vi "Read LIST_IO.vi"(0 "file (use dialog)":path) -> (11 "IP":string, 15 "MERKER":T2, 18 "DATABLOCK":T1)   [LabVIEW 2019]
uses:
  <vilib>/Utility/file.llb/Read Delimited Spreadsheet (string).vi
panel:
  out "all rows":string[][](array[string])
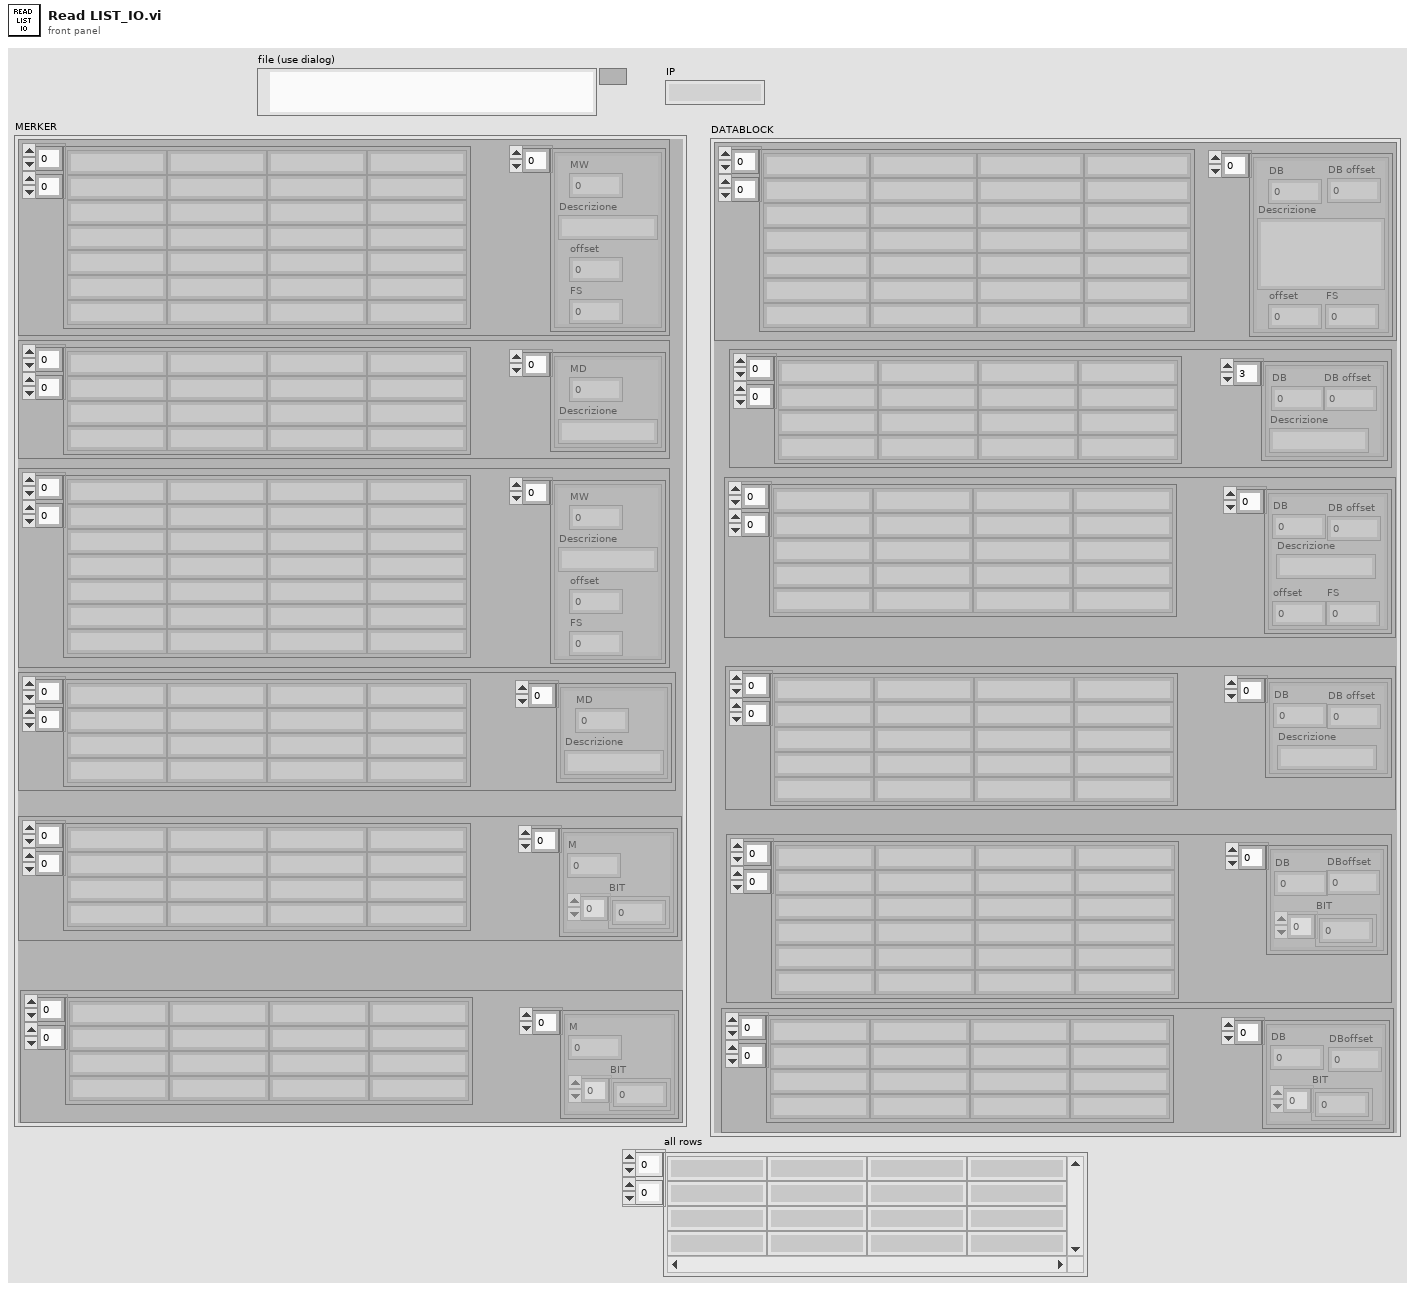
[diagram p1: front panel]
types:
  T1 = cluster{cluster{string[][], cluster{"DB":i16, "DB offset":i16, "Descrizione":string, "offset":dbl, "FS":dbl}[]}, cluster{string[][], cluster{"DB":i16, "Descrizione":string, "DB offset":i16}[]}, cluster{string[][], cluster{"DB":i16, "DB offset":i16, "Descrizione":string, "offset":dbl, "FS":dbl}[]}, cluster{string[][], cluster{"DB":i16, "Descrizione":string, "DB offset":i16}[]}, cluster{string[][], cluster{"DB":i16, "BIT":i16[], "DBoffset":i16}[]}, cluster{string[][], cluster{"DB":i16, "BIT":i16[], "DBoffset":i16}[]}}
  T2 = cluster{cluster{string[][], cluster{"MW":dbl, "Descrizione":string, "offset":dbl, "FS":dbl}[]}, cluster{string[][], cluster{"MD":i16, "Descrizione":string}[]}, cluster{string[][], cluster{"MW":dbl, "Descrizione":string, "offset":dbl, "FS":dbl}[]}, cluster{string[][], cluster{"MD":i16, "Descrizione":string}[]}, cluster{string[][], cluster{"M":i16, "BIT":i16[]}[]}, cluster{string[][], cluster{"M":i16, "BIT":i16[]}[]}}
  T3 = cluster{"DB":i16, "Descrizione":string, "DB offset":i16}
  T4 = cluster{"DB":i16, "DB offset":i16, "Descrizione":string, "offset":dbl, "FS":dbl}
  T5 = cluster{"MW":dbl, "Descrizione":string, "offset":dbl, "FS":dbl}
  T6 = cluster{"DB":i16, "Descrizione":string, "DB offset":i16}[]
  T7 = cluster{string[][], cluster{"MW":dbl, "Descrizione":string, "offset":dbl, "FS":dbl}[]}
  T8 = cluster{string[][], cluster{"MD":i16, "Descrizione":string}[]}
  T9 = cluster{string[][], cluster{"M":i16, "BIT":i16[]}[]}
  T10 = cluster{string[][], cluster{"DB":i16, "BIT":i16[], "DBoffset":i16}[]}
  T11 = cluster{string[][], cluster{"DB":i16, "DB offset":i16, "Descrizione":string, "offset":dbl, "FS":dbl}[]}
  T12 = cluster{string[][], cluster{"DB":i16, "Descrizione":string, "DB offset":i16}[]}
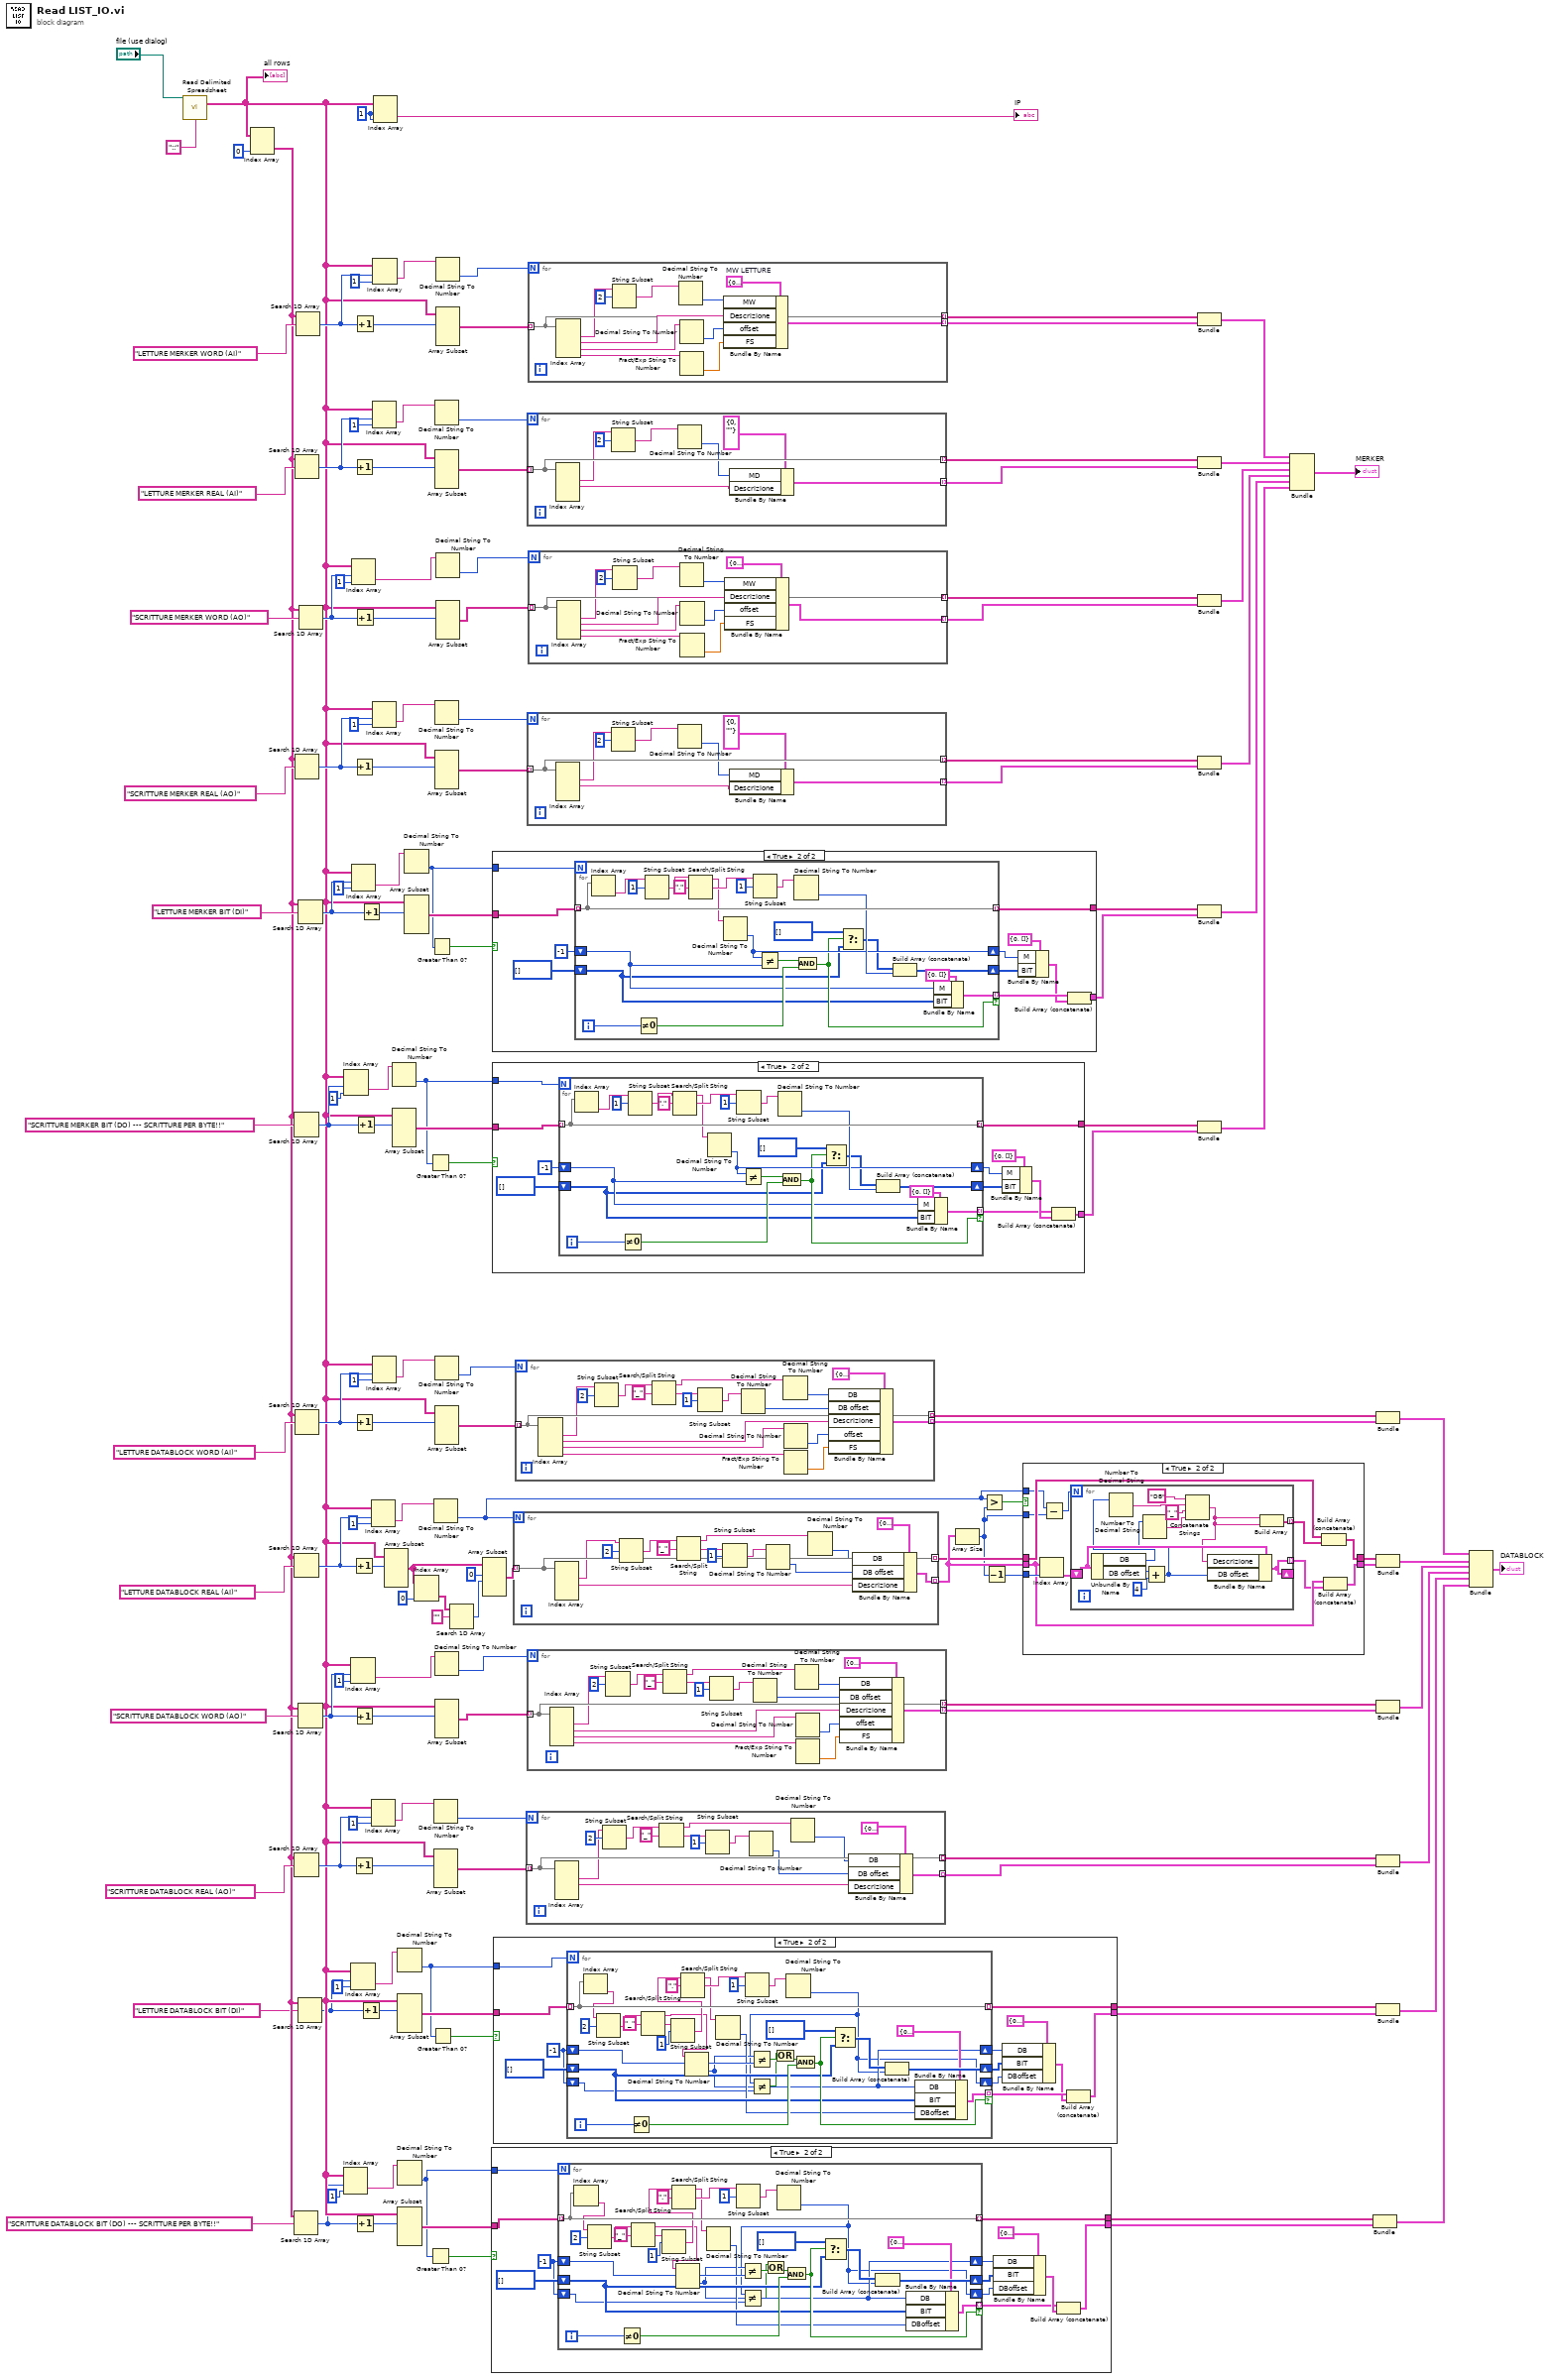
[diagram p0: block diagram]
diagram:
  w115 = 1 ("index (row)")
  n1 = call-poly <vilib>:"Read Delimited Spreadsheet.vi"("file path (dialog if empty)"="file (use dialog)", "delimiter (\\t)"="::" ("delimiter (\\t)")) -> ("all rows"=w45:string[][])  [unwired: 8 in, 5 out]
  "all rows" <- w45
  n2 = Index Array(array=w45, index (col)=0 ("disabled index (col)")) -> (element=w46:string[])  [unwired: 1 in]
  n3 = Search 1D Array(1D array=w46, element="SCRITTURE DATABLOCK BIT (DO) --- SCRITTURE PER BYTE!!") -> (index of element=w36:i32)  [unwired: 1 in]
  n4 = Search 1D Array(1D array=w46, element="SCRITTURE MERKER BIT (DO) --- SCRITTURE PER BYTE!!") -> (index of element=w118:i32)  [unwired: 1 in]
  n5 = Search 1D Array(1D array=w46, element="LETTURE DATABLOCK REAL (AI)") -> (index of element=w62:i32)  [unwired: 1 in]
  n6 = Search 1D Array(1D array=w46, element="SCRITTURE DATABLOCK REAL (AO)") -> (index of element=w65:i32)  [unwired: 1 in]
  n7 = Search 1D Array(1D array=w46, element="LETTURE MERKER REAL (AI)") -> (index of element=w108:i32)  [unwired: 1 in]
  n8 = Search 1D Array(1D array=w46, element="SCRITTURE MERKER REAL (AO)") -> (index of element=w105:i32)  [unwired: 1 in]
  n9 = Search 1D Array(1D array=w46, element="LETTURE DATABLOCK WORD (AI)") -> (index of element=w51:i32)  [unwired: 1 in]
  n10 = Search 1D Array(1D array=w46, element="LETTURE MERKER WORD (AI)") -> (index of element=w133:i32)  [unwired: 1 in]
  n11 = Search 1D Array(1D array=w46, element="LETTURE DATABLOCK BIT (DI)") -> (index of element=w33:i32)  [unwired: 1 in]
  n12 = Search 1D Array(1D array=w46, element="LETTURE MERKER BIT (DI)") -> (index of element=w121:i32)  [unwired: 1 in]
  n13 = Search 1D Array(1D array=w46, element="SCRITTURE DATABLOCK WORD (AO)") -> (index of element=w56:i32)  [unwired: 1 in]
  n14 = Search 1D Array(1D array=w46, element="SCRITTURE MERKER WORD (AO)") -> (index of element=w128:i32)  [unwired: 1 in]
  n15 = Index Array(array=w45, index (row)=w36, index (col)=1 ("disabled index (col)")) -> (element=w35:string)
  n16 = Index Array(array=w45, index (row)=w118, index (col)=1 ("disabled index (col)")) -> (element=w119:string)
  n17 = Index Array(array=w45, index (row)=w56, index (col)=1 ("disabled index (col)")) -> (element=w58:string)
  n18 = Index Array(array=w45, index (row)=w33, index (col)=1 ("disabled index (col)")) -> (element=w31:string)
  n19 = Index Array(array=w45, index (row)=w128, index (col)=1 ("disabled index (col)")) -> (element=w126:string)
  n20 = Index Array(array=w45, index (row)=w121, index (col)=1 ("disabled index (col)")) -> (element=w123:string)
  n21 = Increment(x=w62) -> (x+1=w63:i32)
  n22 = Increment(x=w65) -> (x+1=w64:i32)
  n23 = Increment(x=w108) -> (x+1=w107:i32)
  n24 = Increment(x=w105) -> (x+1=w106:i32)
  n25 = Increment(x=w51) -> (x+1=w54:i32)
  n26 = Increment(x=w56) -> (x+1=w49:i32)
  n27 = Increment(x=w133) -> (x+1=w130:i32)
  n28 = Increment(x=w128) -> (x+1=w140:i32)
  n29 = Increment(x=w36) -> (x+1=w29:i32)
  n30 = Increment(x=w118) -> (x+1=w137:i32)
  n31 = Increment(x=w33) -> (x+1=w34:i32)
  n32 = Increment(x=w121) -> (x+1=w120:i32)
  n33 = Index Array(array=w45, index (row)=w62, index (col)=1 ("disabled index (row)")) -> (element=w60:string)
  n34 = Index Array(array=w45, index (row)=w65, index (col)=1 ("disabled index (row)")) -> (element=w67:string)
  n35 = Index Array(array=w45, index (row)=w108, index (col)=1 ("disabled index (row)")) -> (element=w110:string)
  n36 = Index Array(array=w45, index (row)=w105, index (col)=1 ("disabled index (row)")) -> (element=w103:string)
  n37 = Index Array(array=w45, index (row)=w51, index (col)=1 ("disabled index (row)")) -> (element=w50:string)
  n38 = Index Array(array=w45, index (row)=w133, index (col)=1 ("disabled index (row)")) -> (element=w134:string)
  n39 = Index Array(array=w45, index (row)=w115, index (col)=w115) -> (element=→"IP":string)
  n40 = Array Subset(array=w45, index (row)=w63) -> (w5:string[][])  [unwired: 3 in]
  n41 = Decimal String To Number(string=w119) -> (number=w21:i32)  [unwired: 2 in, 1 out]
  n42 = Array Subset(array=w45, index (row)=w137) -> (w116:string[][])  [unwired: 3 in]
  n43 = Decimal String To Number(string=w31) -> (number=w18:i32)  [unwired: 2 in, 1 out]
  n44 = Array Subset(array=w45, index (row)=w34) -> (w28:string[][])  [unwired: 3 in]
  n45 = Decimal String To Number(string=w35) -> (number=w17:i32)  [unwired: 2 in, 1 out]
  n46 = Array Subset(array=w45, index (row)=w29) -> (w24:string[][])  [unwired: 3 in]
  n47 = Decimal String To Number(string=w123) -> (number=w22:i32)  [unwired: 2 in, 1 out]
  n48 = Array Subset(array=w45, index (row)=w120) -> (w138:string[][])  [unwired: 3 in]
  n49 = Index Array(array=w5, index (col)=0 ("disabled index (col)")) -> (element=w8:string[])  [unwired: 1 in]
  n50 = Greater Than 0?(x=w21) -> (x > 0?=w20:bool)
  n51 = Greater Than 0?(x=w17) -> (x > 0?=w16:bool)
  n52 = Greater Than 0?(x=w22) -> (x > 0?=w23:bool)
  n53 = Greater Than 0?(x=w18) -> (x > 0?=w19:bool)
  n54 = Decimal String To Number(string=w60) -> (number=w10:i32)  [unwired: 2 in, 1 out]
  n55 = Decimal String To Number(string=w67) -> (number=w69:i32)  [unwired: 2 in, 1 out]
  n56 = Array Subset(array=w45, index (row)=w64) -> (w70:string[][])  [unwired: 3 in]
  n57 = Decimal String To Number(string=w110) -> (number=w112:i32)  [unwired: 2 in, 1 out]
  n58 = Array Subset(array=w45, index (row)=w107) -> (w113:string[][])  [unwired: 3 in]
  n59 = Decimal String To Number(string=w103) -> (number=w101:i32)  [unwired: 2 in, 1 out]
  n60 = Array Subset(array=w45, index (row)=w106) -> (w100:string[][])  [unwired: 3 in]
  n61 = Decimal String To Number(string=w50) -> (number=w53:i32)  [unwired: 2 in, 1 out]
  n62 = Array Subset(array=w45, index (row)=w54) -> (w55:string[][])  [unwired: 3 in]
  n63 = Decimal String To Number(string=w58) -> (number=w44:i32)  [unwired: 2 in, 1 out]
  n64 = Array Subset(array=w45, index (row)=w49) -> (w43:string[][])  [unwired: 3 in]
  n65 = Decimal String To Number(string=w134) -> (number=w131:i32)  [unwired: 2 in, 1 out]
  n66 = Array Subset(array=w45, index (row)=w130) -> (w129:string[][])  [unwired: 3 in]
  n67 = Decimal String To Number(string=w126) -> (number=w124:i32)  [unwired: 2 in, 1 out]
  n68 = Array Subset(array=w45, index (row)=w140) -> (w125:string[][])  [unwired: 3 in]
  n69 = Search 1D Array(1D array=w8, element="") -> (index of element=w2:i32)  [unwired: 1 in]
  n70 = Array Subset(array=w5, index (row)=0 ("index"), length (row)=w2) -> (w4:string[][])  [unwired: 2 in]
  n71 = case shown="True" w16 {
    tunnel: [_ w151] -> w26
    tunnel: [_ w150] -> w25
    tunnel: w17 -> [_ w149]
    tunnel: w24 -> [_ w148]
    frame False {
    }
    frame True {
      w147 = -1 ("offset past number")
      n72 = for {
        N: w149 -> [_]
        tunnel: w148 -> [w187] mode=indexing
        tunnel: [w187] -> w151 mode=indexing
        shift-right: [w161] -> w155
        shift-left: w147 -> [w176]
        shift-right: [w174] -> w146
        shift-left: i32[] [] ("BIT") -> [w173]
        tunnel: [w181] -> w152 mode=indexing if=w179
        shift-right: [w159] -> w145
        shift-left: w147 -> [w160]
        i -> [w177]
        n73 = Index Array(array=w187) -> (element=w166:string)  [unwired: 1 in]
        n74 = String Subset(string=w166, offset (0)=2) -> (substring=w171:string)  [unwired: 1 in]
        n75 = Not Equal To 0?(x=w177) -> (x != 0?=w178:bool)
        n76 = Search/Split String(string=w171, search string/char (-)="_") -> (substring before match=w162:string, match + rest of string=w169:string)  [unwired: 1 in, 1 out]
        n77 = String Subset(string=w169, offset (0)=1) -> (substring=w165:string)  [unwired: 1 in]
        n78 = Search/Split String(string=w165, search string/char (-)=".") -> (substring before match=w182:string, match + rest of string=w184:string)  [unwired: 1 in, 1 out]
        n79 = Decimal String To Number(string=w162) -> (number=w161:i32)  [unwired: 2 in, 1 out]
        n80 = Decimal String To Number(string=w182) -> (number=w163:i32)  [unwired: 2 in, 1 out]
        n81 = String Subset(string=w184, offset (0)=1) -> (substring=w183:string)  [unwired: 1 in]
        n82 = Not Equal?(x=w161, y=w176) -> (x != y?=w175:bool)
        n83 = Decimal String To Number(string=w183) -> (number=w159:i32)  [unwired: 2 in, 1 out]
        n84 = Not Equal?(x=w159, y=w160) -> (x != y?=w157:bool)
        n85 = Or(x=w157, y=w175) -> (x .or. y?=w158:bool)
        n86 = And(x=w158, y=w178) -> (x .and. y?=w179:bool)
        n87 = Select(t=i16[] [] ("BIT"), s=w179, f=w173) -> (s? t:f=w172:i32[])
        n88 = Build Array (concatenate)(w172, w159) -> (w174:i32[])
        n89 = Bundle By Name(cluster=cluster{"DB":i16, "BIT":i16[], "DBoffset":i16} {"DB"=0, "BIT"=[], "DBoffset"=0} ("M BIT LETTURE"), "DB"=w161, "BIT"=w173, "DBoffset"=w163) -> (w181:cluster{"DB":i16, "BIT":i16[], "DBoffset":i16})
      }
      n90 = Bundle By Name(cluster=cluster{"DB":i16, "BIT":i16[], "DBoffset":i16} {"DB"=0, "BIT"=[], "DBoffset"=0} ("M BIT LETTURE"), "DB"=w155, "BIT"=w146, "DBoffset"=w145) -> (w156:cluster{"DB":i16, "BIT":i16[], "DBoffset":i16})
      n91 = Build Array (concatenate)(w152, w156) -> (w150:cluster{"DB":i16, "BIT":i16[], "DBoffset":i16}[])
    }
  }
  n92 = case shown="True" w23 {
    tunnel: w138 -> [_ w198]
    tunnel: w22 -> [_ w197]
    tunnel: [_ w189] -> w91
    tunnel: [_ w188] -> w90
    frame False {
    }
    frame True {
      n93 = for {
        N: w197 -> [_]
        tunnel: w198 -> [w220] mode=indexing
        tunnel: [w220] -> w189 mode=indexing
        shift-right: [w207] -> w193
        shift-left: -1 ("offset past number") -> [w203]
        shift-right: [w201] -> w192
        shift-left: i32[] [] ("BIT") -> [w200]
        tunnel: [w210] -> w191 mode=indexing if=w206
        i -> [w204]
        n94 = Index Array(array=w220) -> (element=w218:string)  [unwired: 1 in]
        n95 = Not Equal To 0?(x=w204) -> (x != 0?=w205:bool)
        n96 = String Subset(string=w218, offset (0)=1) -> (substring=w216:string)  [unwired: 1 in]
        n97 = Search/Split String(string=w216, search string/char (-)=".") -> (substring before match=w212:string, match + rest of string=w214:string)  [unwired: 1 in, 1 out]
        n98 = Decimal String To Number(string=w212) -> (number=w207:i32)  [unwired: 2 in, 1 out]
        n99 = String Subset(string=w214, offset (0)=1) -> (substring=w213:string)  [unwired: 1 in]
        n100 = Not Equal?(x=w207, y=w203) -> (x != y?=w202:bool)
        n101 = Decimal String To Number(string=w213) -> (number=w208:i32)  [unwired: 2 in, 1 out]
        n102 = And(x=w202, y=w205) -> (x .and. y?=w206:bool)
        n103 = Select(t=i16[] [] ("BIT"), s=w206, f=w200) -> (s? t:f=w199:i32[])
        n104 = Build Array (concatenate)(w199, w208) -> (w201:i32[])
        n105 = Bundle By Name(cluster=cluster{"M":i16, "BIT":i16[]} {"M"=0, "BIT"=[]} ("M BIT LETTURE"), "M"=w203, "BIT"=w200) -> (w210:cluster{"M":i16, "BIT":i16[]})
      }
      n106 = Bundle By Name(cluster=cluster{"M":i16, "BIT":i16[]} {"M"=0, "BIT"=[]} ("M BIT LETTURE"), "M"=w193, "BIT"=w192) -> (w190:cluster{"M":i16, "BIT":i16[]})
      n107 = Build Array (concatenate)(w191, w190) -> (w188:cluster{"M":i16, "BIT":i16[]}[])
    }
  }
  n108 = case shown="True" w20 {
    tunnel: w21 -> [_ w224]
    tunnel: w116 -> [_ w223]
    tunnel: [_ w222] -> w89
    tunnel: [_ w221] -> w88
    frame False {
    }
    frame True {
      n109 = for {
        N: w224 -> [_]
        tunnel: w223 -> [w253] mode=indexing
        tunnel: [w253] -> w222 mode=indexing
        shift-right: [w240] -> w228
        shift-left: -1 ("offset past number") -> [w236]
        shift-right: [w234] -> w229
        shift-left: i32[] [] ("BIT") -> [w233]
        tunnel: [w243] -> w230 mode=indexing if=w239
        i -> [w237]
        n110 = Index Array(array=w253) -> (element=w251:string)  [unwired: 1 in]
        n111 = Not Equal To 0?(x=w237) -> (x != 0?=w238:bool)
        n112 = String Subset(string=w251, offset (0)=1) -> (substring=w249:string)  [unwired: 1 in]
        n113 = Search/Split String(string=w249, search string/char (-)=".") -> (substring before match=w245:string, match + rest of string=w247:string)  [unwired: 1 in, 1 out]
        n114 = Decimal String To Number(string=w245) -> (number=w240:i32)  [unwired: 2 in, 1 out]
        n115 = String Subset(string=w247, offset (0)=1) -> (substring=w246:string)  [unwired: 1 in]
        n116 = Not Equal?(x=w240, y=w236) -> (x != y?=w235:bool)
        n117 = Decimal String To Number(string=w246) -> (number=w241:i32)  [unwired: 2 in, 1 out]
        n118 = And(x=w235, y=w238) -> (x .and. y?=w239:bool)
        n119 = Select(t=i16[] [] ("BIT"), s=w239, f=w233) -> (s? t:f=w232:i32[])
        n120 = Build Array (concatenate)(w232, w241) -> (w234:i32[])
        n121 = Bundle By Name(cluster=cluster{"M":i16, "BIT":i16[]} {"M"=0, "BIT"=[]} ("M BIT LETTURE"), "M"=w236, "BIT"=w233) -> (w243:cluster{"M":i16, "BIT":i16[]})
      }
      n122 = Bundle By Name(cluster=cluster{"M":i16, "BIT":i16[]} {"M"=0, "BIT"=[]} ("M BIT LETTURE"), "M"=w228, "BIT"=w229) -> (w231:cluster{"M":i16, "BIT":i16[]})
      n123 = Build Array (concatenate)(w230, w231) -> (w221:cluster{"M":i16, "BIT":i16[]}[])
    }
  }
  n124 = case shown="True" w19 {
    tunnel: [_ w265] -> w39
    tunnel: [_ w264] -> w38
    tunnel: w18 -> [_ w261]
    tunnel: w28 -> [_ w260]
    frame False {
    }
    frame True {
      w259 = -1 ("offset past number")
      n125 = for {
        N: w261 -> [_]
        tunnel: w260 -> [w296] mode=indexing
        tunnel: [w296] -> w264 mode=indexing
        shift-right: [w270] -> w257
        shift-left: w259 -> [w285]
        shift-right: [w283] -> w256
        shift-left: i32[] [] ("BIT") -> [w282]
        tunnel: [w290] -> w263 mode=indexing if=w288
        shift-right: [w268] -> w255
        shift-left: w259 -> [w269]
        i -> [w286]
        n126 = Index Array(array=w296) -> (element=w275:string)  [unwired: 1 in]
        n127 = String Subset(string=w275, offset (0)=2) -> (substring=w280:string)  [unwired: 1 in]
        n128 = Not Equal To 0?(x=w286) -> (x != 0?=w287:bool)
        n129 = Search/Split String(string=w280, search string/char (-)="_") -> (substring before match=w271:string, match + rest of string=w278:string)  [unwired: 1 in, 1 out]
        n130 = String Subset(string=w278, offset (0)=1) -> (substring=w274:string)  [unwired: 1 in]
        n131 = Search/Split String(string=w274, search string/char (-)=".") -> (substring before match=w291:string, match + rest of string=w293:string)  [unwired: 1 in, 1 out]
        n132 = Decimal String To Number(string=w271) -> (number=w270:i32)  [unwired: 2 in, 1 out]
        n133 = Decimal String To Number(string=w291) -> (number=w272:i32)  [unwired: 2 in, 1 out]
        n134 = String Subset(string=w293, offset (0)=1) -> (substring=w292:string)  [unwired: 1 in]
        n135 = Not Equal?(x=w270, y=w285) -> (x != y?=w284:bool)
        n136 = Decimal String To Number(string=w292) -> (number=w268:i32)  [unwired: 2 in, 1 out]
        n137 = Not Equal?(x=w268, y=w269) -> (x != y?=w266:bool)
        n138 = Or(x=w266, y=w284) -> (x .or. y?=w267:bool)
        n139 = And(x=w267, y=w287) -> (x .and. y?=w288:bool)
        n140 = Select(t=i16[] [] ("BIT"), s=w288, f=w282) -> (s? t:f=w281:i32[])
        n141 = Build Array (concatenate)(w281, w268) -> (w283:i32[])
        n142 = Bundle By Name(cluster=cluster{"DB":i16, "BIT":i16[], "DBoffset":i16} {"DB"=0, "BIT"=[], "DBoffset"=0} ("M BIT LETTURE"), "DB"=w270, "BIT"=w282, "DBoffset"=w272) -> (w290:cluster{"DB":i16, "BIT":i16[], "DBoffset":i16})
      }
      n143 = Bundle By Name(cluster=cluster{"DB":i16, "BIT":i16[], "DBoffset":i16} {"DB"=0, "BIT"=[], "DBoffset"=0} ("M BIT LETTURE"), "DB"=w257, "BIT"=w256, "DBoffset"=w255) -> (w254:cluster{"DB":i16, "BIT":i16[], "DBoffset":i16})
      n144 = Build Array (concatenate)(w263, w254) -> (w265:cluster{"DB":i16, "BIT":i16[], "DBoffset":i16}[])
    }
  }
  n145 = for {
    N: w10 -> [_]
    tunnel: [w310] -> w12 mode=indexing
    tunnel: w4 -> [w310] mode=indexing
    tunnel: [w308] -> w14 mode=indexing
    n146 = Index Array(array=w310) -> (element #1=w299:string, element #2=w309:string)  [unwired: 4 in, 2 out]
    n147 = String Subset(string=w299, offset (0)=2) -> (substring=w301:string)  [unwired: 1 in]
    n148 = Search/Split String(string=w301, search string/char (-)="_") -> (substring before match=w302:string, match + rest of string=w304:string)  [unwired: 1 in, 1 out]
    n149 = String Subset(string=w304, offset (0)=1) -> (substring=w306:string)  [unwired: 1 in]
    n150 = Decimal String To Number(string=w306) -> (number=w297:i32)  [unwired: 2 in, 1 out]
    n151 = Decimal String To Number(string=w302) -> (number=w298:i32)  [unwired: 2 in, 1 out]
    n152 = Bundle By Name(cluster=T3 {"DB"=0, "Descrizione"="", "DB offset"=0} ("MW LETTURE 2"), "DB"=w298, "DB offset"=w297, "Descrizione"=w309) -> (w308:T3)
  }
  n153 = for {
    N: w53 -> [_]
    tunnel: [w322] -> w71 mode=indexing
    tunnel: [w323] -> w72 mode=indexing
    tunnel: w55 -> [w322] mode=indexing
    n154 = Index Array(array=w322) -> (element #1=w321:string, element #2=w328:string, element #3=w327:string, element #4=w325:string)  [unwired: 4 in]
    n155 = String Subset(string=w321, offset (0)=2) -> (substring=w319:string)  [unwired: 1 in]
    n156 = Search/Split String(string=w319, search string/char (-)="_") -> (substring before match=w318:string, match + rest of string=w316:string)  [unwired: 1 in, 1 out]
    n157 = String Subset(string=w316, offset (0)=1) -> (substring=w314:string)  [unwired: 1 in]
    n158 = Decimal String To Number(string=w314) -> (number=w312:i32)  [unwired: 2 in, 1 out]
    n159 = Decimal String To Number(string=w318) -> (number=w313:i32)  [unwired: 2 in, 1 out]
    n160 = Decimal String To Number(string=w327) -> (number=w326:i32)  [unwired: 2 in, 1 out]
    n161 = Fract/Exp String To Number(string=w325) -> (number=w324:dbl)  [unwired: 3 in, 1 out]
    n162 = Bundle By Name(cluster=T4 {"DB"=0, "DB offset"=0, "Descrizione"="", "offset"=0.0, "FS"=0.0} ("MW LETTURE 2"), "DB"=w313, "DB offset"=w312, "Descrizione"=w328, "offset"=w326, "FS"=w324) -> (w323:T4)
  }
  n163 = for {
    N: w69 -> [_]
    tunnel: [w342] -> w73 mode=indexing
    tunnel: w70 -> [w342] mode=indexing
    tunnel: [w340] -> w74 mode=indexing
    n164 = Index Array(array=w342) -> (element #1=w332:string, element #2=w341:string)  [unwired: 4 in, 2 out]
    n165 = String Subset(string=w332, offset (0)=2) -> (substring=w334:string)  [unwired: 1 in]
    n166 = Search/Split String(string=w334, search string/char (-)="_") -> (substring before match=w335:string, match + rest of string=w337:string)  [unwired: 1 in, 1 out]
    n167 = String Subset(string=w337, offset (0)=1) -> (substring=w339:string)  [unwired: 1 in]
    n168 = Decimal String To Number(string=w339) -> (number=w329:i32)  [unwired: 2 in, 1 out]
    n169 = Decimal String To Number(string=w335) -> (number=w330:i32)  [unwired: 2 in, 1 out]
    n170 = Bundle By Name(cluster=T3 {"DB"=0, "Descrizione"="", "DB offset"=0} ("MW LETTURE 2"), "DB"=w330, "DB offset"=w329, "Descrizione"=w341) -> (w340:T3)
  }
  n171 = for {
    N: w112 -> [_]
    tunnel: [w350] -> w97 mode=indexing
    tunnel: w113 -> [w350] mode=indexing
    tunnel: [w343] -> w96 mode=indexing
    n172 = Index Array(array=w350) -> (element #1=w349:string, element #2=w344:string)  [unwired: 4 in, 2 out]
    n173 = String Subset(string=w349, offset (0)=2) -> (substring=w347:string)  [unwired: 1 in]
    n174 = Decimal String To Number(string=w347) -> (number=w345:i32)  [unwired: 2 in, 1 out]
    n175 = Bundle By Name(cluster=cluster{"MD":i16, "Descrizione":string} {"MD"=0, "Descrizione"=""} ("MW LETTURE 2"), "MD"=w345, "Descrizione"=w344) -> (w343:cluster{"MD":i16, "Descrizione":string})
  }
  n176 = for {
    N: w101 -> [_]
    tunnel: [w358] -> w93 mode=indexing
    tunnel: w100 -> [w358] mode=indexing
    tunnel: [w351] -> w92 mode=indexing
    n177 = Index Array(array=w358) -> (element #1=w357:string, element #2=w352:string)  [unwired: 4 in, 2 out]
    n178 = String Subset(string=w357, offset (0)=2) -> (substring=w355:string)  [unwired: 1 in]
    n179 = Decimal String To Number(string=w355) -> (number=w353:i32)  [unwired: 2 in, 1 out]
    n180 = Bundle By Name(cluster=cluster{"MD":i16, "Descrizione":string} {"MD"=0, "Descrizione"=""} ("MW LETTURE 2"), "MD"=w353, "Descrizione"=w352) -> (w351:cluster{"MD":i16, "Descrizione":string})
  }
  n181 = for {
    N: w44 -> [_]
    tunnel: [w370] -> w42 mode=indexing
    tunnel: [w371] -> w41 mode=indexing
    tunnel: w43 -> [w370] mode=indexing
    n182 = Index Array(array=w370) -> (element #1=w369:string, element #2=w376:string, element #3=w375:string, element #4=w373:string)  [unwired: 4 in]
    n183 = String Subset(string=w369, offset (0)=2) -> (substring=w367:string)  [unwired: 1 in]
    n184 = Search/Split String(string=w367, search string/char (-)="_") -> (substring before match=w366:string, match + rest of string=w364:string)  [unwired: 1 in, 1 out]
    n185 = String Subset(string=w364, offset (0)=1) -> (substring=w362:string)  [unwired: 1 in]
    n186 = Decimal String To Number(string=w362) -> (number=w360:i32)  [unwired: 2 in, 1 out]
    n187 = Decimal String To Number(string=w366) -> (number=w361:i32)  [unwired: 2 in, 1 out]
    n188 = Decimal String To Number(string=w375) -> (number=w374:i32)  [unwired: 2 in, 1 out]
    n189 = Fract/Exp String To Number(string=w373) -> (number=w372:dbl)  [unwired: 3 in, 1 out]
    n190 = Bundle By Name(cluster=T4 {"DB"=0, "DB offset"=0, "Descrizione"="", "offset"=0.0, "FS"=0.0} ("MW LETTURE 2"), "DB"=w361, "DB offset"=w360, "Descrizione"=w376, "offset"=w374, "FS"=w372) -> (w371:T4)
  }
  n191 = for {
    N: w131 -> [_]
    tunnel: [w380] -> w99 mode=indexing
    tunnel: [w381] -> w98 mode=indexing
    tunnel: w129 -> [w380] mode=indexing
    w388 = T5 {"MW"=0.0, "Descrizione"="", "offset"=0.0, "FS"=0.0}  # MW LETTURE
    n192 = Index Array(array=w380) -> (element #1=w379:string, element #2=w386:string, element #3=w385:string, element #4=w383:string)  [unwired: 4 in]
    n193 = String Subset(string=w379, offset (0)=2) -> (substring=w377:string)  [unwired: 1 in]
    n194 = Decimal String To Number(string=w377) -> (number=w387:i32)  [unwired: 2 in, 1 out]
    n195 = Decimal String To Number(string=w385) -> (number=w384:i32)  [unwired: 2 in, 1 out]
    n196 = Fract/Exp String To Number(string=w383) -> (number=w382:dbl)  [unwired: 3 in, 1 out]
    n197 = Bundle By Name(cluster=w388, "MW"=w387, "Descrizione"=w386, "offset"=w384, "FS"=w382) -> (w381:T5)
  }
  n198 = for {
    N: w124 -> [_]
    tunnel: [w392] -> w95 mode=indexing
    tunnel: [w393] -> w94 mode=indexing
    tunnel: w125 -> [w392] mode=indexing
    n199 = Index Array(array=w392) -> (element #1=w391:string, element #2=w398:string, element #3=w397:string, element #4=w395:string)  [unwired: 4 in]
    n200 = String Subset(string=w391, offset (0)=2) -> (substring=w389:string)  [unwired: 1 in]
    n201 = Decimal String To Number(string=w389) -> (number=w399:i32)  [unwired: 2 in, 1 out]
    n202 = Decimal String To Number(string=w397) -> (number=w396:i32)  [unwired: 2 in, 1 out]
    n203 = Fract/Exp String To Number(string=w395) -> (number=w394:dbl)  [unwired: 3 in, 1 out]
    n204 = Bundle By Name(cluster=T5 {"MW"=0.0, "Descrizione"="", "offset"=0.0, "FS"=0.0} ("MW LETTURE"), "MW"=w399, "Descrizione"=w398, "offset"=w396, "FS"=w394) -> (w393:T5)
  }
  n205 = Array Size(array=w14) -> (size(s)=w9:i32)
  n206 = Greater?(x=w10, y=w9) -> (0:w15:bool)
  n207 = Decrement(x=w9) -> (x-1=w1:i32)
  n208 = case shown="True" w15 {
    tunnel: w14 -> [w401 w411]
    tunnel: w1 -> [_ w413]
    tunnel: [w401 w409] -> w13
    tunnel: w12 -> [w402 w408]
    tunnel: [w402 w406] -> w11
    tunnel: w10 -> [_ w405]
    tunnel: w9 -> [_ w404]
    frame False {
    }
    frame True {
      n209 = Index Array(array=w411, index=w413) -> (element=w412:T3)
      n210 = Subtract(x=w405, y=w404) -> (x-y=w403:i32)
      n211 = for {
        N: w403 -> [_]
        shift-right: [w417] -> _
        shift-left: w412 -> [w425]
        tunnel: [w416] -> w407 mode=indexing
        tunnel: [w417] -> w410 mode=indexing
        n212 = Unbundle By Name(w425) -> ("DB"=w423:i16, "DB offset"=w419:i16)
        n213 = Number To Decimal String(number=w423) -> (decimal integer string=w422:string)  [unwired: 1 in]
        n214 = Add(x=w419, y=i16 4) -> (x+y=w415:i16)
        n215 = Number To Decimal String(number=w415) -> (decimal integer string=w418:string)  [unwired: 1 in]
        n216 = Concatenate Strings("DB" ("string"), w422, "_" ("string"), w418) -> (w414:string)
        n217 = Bundle By Name(cluster=w425, "Descrizione"=w414, "DB offset"=w415) -> (w417:T3)
        n218 = Build Array(w414, w414) -> (w416:string[])
      }
      n219 = Build Array (concatenate)(w408, w407) -> (w406:string[][])
      n220 = Build Array (concatenate)(w411, w410) -> (w409:T6)
    }
  }
  n221 = Bundle(w99, w98) -> (w87:T7)  [unwired: 1 in]
  n222 = Bundle(w97, w96) -> (w86:T8)  [unwired: 1 in]
  n223 = Bundle(w95, w94) -> (w85:T7)  [unwired: 1 in]
  n224 = Bundle(w93, w92) -> (w84:T8)  [unwired: 1 in]
  n225 = Bundle(w91, w90) -> (w83:T9)  [unwired: 1 in]
  n226 = Bundle(w89, w88) -> (w82:T9)  [unwired: 1 in]
  n227 = Bundle(w87, w86, w85, w84, w83, w82) -> (→"MERKER":T2)  [unwired: 1 in]
  n228 = Bundle(w26, w25) -> (w80:T10)  [unwired: 1 in]
  n229 = Bundle(w71, w72) -> (w75:T11)  [unwired: 1 in]
  n230 = Bundle(w11, w13) -> (w76:T12)  [unwired: 1 in]
  n231 = Bundle(w42, w41) -> (w77:T11)  [unwired: 1 in]
  n232 = Bundle(w73, w74) -> (w78:T12)  [unwired: 1 in]
  n233 = Bundle(w38, w39) -> (w79:T10)  [unwired: 1 in]
  n234 = Bundle(w75, w76, w77, w78, w79, w80) -> (→"DATABLOCK":T1)  [unwired: 1 in]
